vi "Main.vi"() -> ()   [LabVIEW 2015]
uses:
  Globals.vi
panel:
  in  "Slide":dbl(slide) scale=0.0..10.0
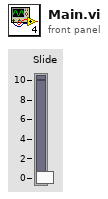
[diagram p1: front panel]
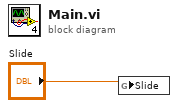
[diagram p0: block diagram]
diagram:
  n1 = global write "Globals.vi" "Slide"("Slide") -> ()
